vi "camera_closer.vi"(0 "input cluster":T2) -> ()   [LabVIEW 2010]
uses:
  <vilib>/userDefined/High Color/IMAQdx.ctl
  <vilib>/vision/driver/NI_Vision_Acquisition_Software.lvlib
  Image-Stack-Compressor/Stack Reader Wrapper/labview vis/StackReaderWrapper.lvlib
panel:
  out "mmf error out":errorcluster
  out "AVI error out":errorcluster
  out "IMAQdx error out":errorcluster
  out "IMAQ error out":errorcluster
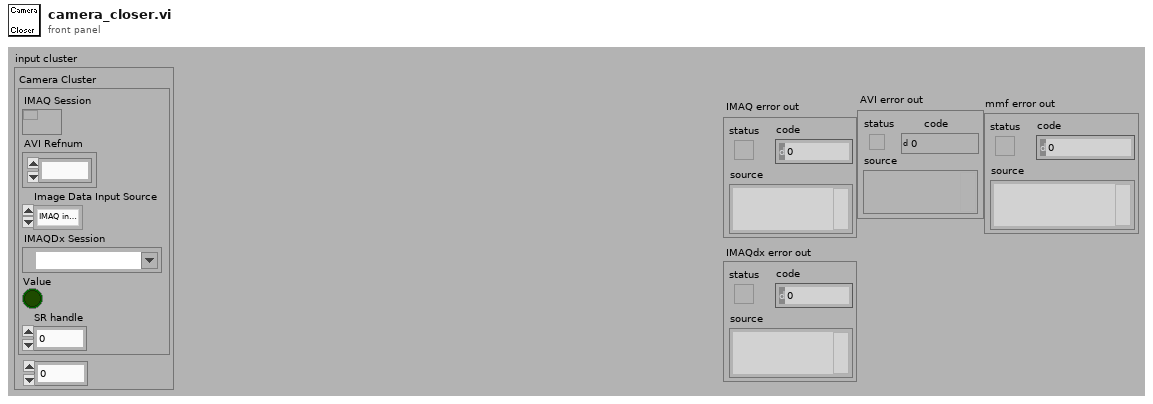
[diagram p1: front panel]
types:
  T1 = typedef "IMAQdx.ctl" = refnum<k21>
  T2 = cluster{"Camera Cluster":cluster{"IMAQ Session":refnum<k11>, "AVI Refnum":refnum<k1>, "Image Data Input Source":enum32{"IMAQ interface", "IMAQdx interface", "AVI file", "MMF File"}, "IMAQDx Session":T1, "Value":bool, "SR handle":u32}, i32}
  T3 = cluster{"IMAQ Session":refnum<k11>, "AVI Refnum":refnum<k1>, "Image Data Input Source":enum32{"IMAQ interface", "IMAQdx interface", "AVI file", "MMF File"}, "IMAQDx Session":T1, "Value":bool, "SR handle":u32}
  T4 = enum32{"IMAQ interface", "IMAQdx interface", "AVI file", "MMF File"}
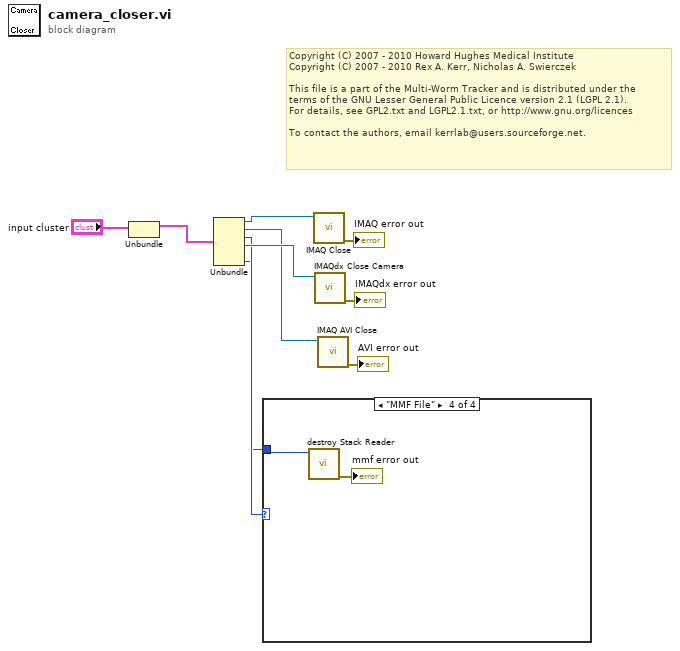
[diagram p0: block diagram]
diagram:
  # "Copyright (C) 2007 - 2010 Howard Hughes Medical Institute\nCopyright (C) 2007 - 2010 Rex A. Kerr, Nicholas A. Swierczek\n \nThis file is a part of the Multi-Worm Tracker and is distributed under the\nterms of the GNU Lesser General Public Licence version 2.1 (LGPL 2.1).\nFor details, see GPL2.txt and LGPL2.1.txt, or http://www.gnu.org/licences\n \nTo contact the authors, email kerrlab@users.sourceforge.net."
  n1 = Unbundle("input cluster") -> ("Camera Cluster"=w10:T3)  [unwired: 1 out]
  n2 = Unbundle(w10) -> ("IMAQ Session"=w9:refnum<k11>, "AVI Refnum"=w4:refnum<k1>, "Image Data Input Source"=w2:T4, "IMAQDx Session"=w5:T1, "SR handle"=w1:u32)  [unwired: 1 out]
  n3 = case shown="\"MMF File\"" w2 {
    tunnel: w1 -> [_ _ _ w12]
    frame "IMAQ interface", Default {
    }
    frame "IMAQdx interface" {
    }
    frame "AVI file" {
    }
    frame "MMF File" {
      n4 = call "destroy Stack Reader.vi"("sr"=w12) -> ("error out"=→"mmf error out":errorcluster)  [unwired: 9 in, 1 out]
    }
  }
  n5 = call <vilib>:"IMAQ Close.vi"("IMAQ Session In"=w9) -> ("error out"=→"IMAQ error out":errorcluster)  [unwired: 10 in]
  n6 = call <vilib>:"IMAQdx Close Camera.vi"("Session In"=w5) -> ("error out"=→"IMAQdx error out":errorcluster)  [unwired: 10 in]
  n7 = call "IMAQ AVI Close"("Avi Refnum"=w4) -> ("error out"=→"AVI error out":errorcluster)  [unwired: 10 in]
